vi "Initialize From Settings.vi"(8 "error in (no error)":errorcluster, 10 "settings":cluster{"key":string, "value":string}[](array[cluster]), 11 "Core Groups Configuration in":refnum<class "Group Configuration.lvclass">) -> (0 "error out":errorcluster, 3 "Core Groups Configuration out":refnum<class "Group Configuration.lvclass">)   [LabVIEW 2021, in "DSF Core.lvlib" / "Group Configuration.lvclass"]
uses:
  Group Configuration.lvclass
  Group Configuration.lvclass/Group Configuration.ctl
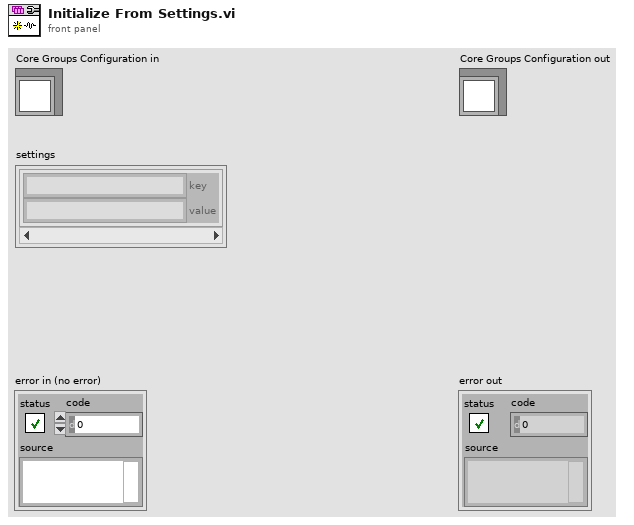
[diagram p1: front panel]
types:
  T1 = cluster{"name":string, "direction":enum8{"Tx", "Rx"}, "cycle timing":cluster{"priority":u64, "decimation":u64, "offset":u64}, "timeout behavior":enum8{"Increment Late Count", "Throw Error"}, "enable conversion":bool}
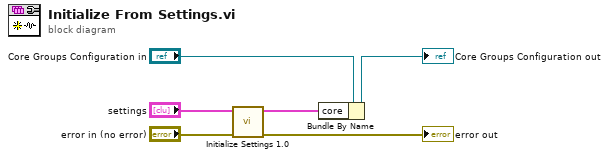
[diagram p0: block diagram]
diagram:
  n1 = call "Initialize Settings 1.0.vi"("error in (no error)"="error in (no error)", "settings 1.0"="settings") -> ("error out"=→"error out":errorcluster, "configuration 1.0"=w4:T1)  [unwired: 8 in]
  n2 = Bundle By Name(cluster="Core Groups Configuration in", "core"=w4) -> (→"Core Groups Configuration out":refnum<class "Group Configuration.lvclass">)
